vi "TypeCheck.vi"(11 "Variant in":variant) -> (2 "DbType":i32, 3 "Variant out":variant)   [LabVIEW 2020, in "ORM.lvlib" / "DbConnection.lvclass"]
uses:
  DbConnection.lvclass
  <vilib>/regexp/Match Regular Expression.xnode
  DbConnection.lvclass/DbConnection.ctl
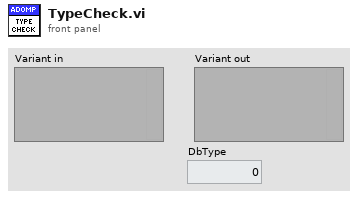
[diagram p1: front panel]
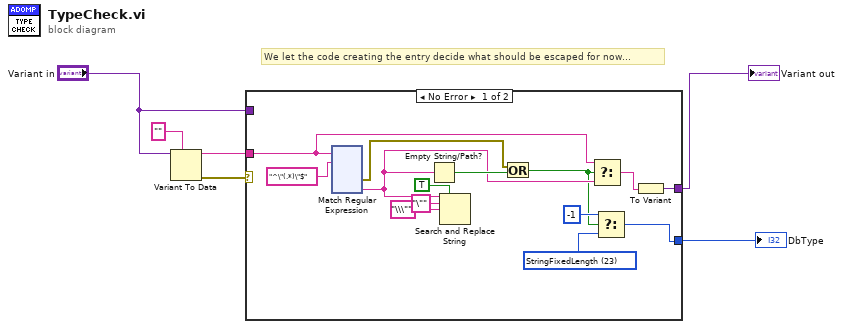
[diagram p0: block diagram]
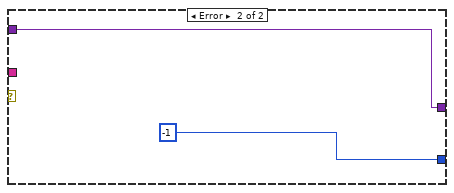
[diagram p2: hidden frame]
diagram:
  # "We let the code creating the entry decide what should be escaped for now..."
  n1 = Variant To Data(type="", Variant="Variant in") -> (data=w4:string, error out=w5:errorcluster)  [unwired: 1 in]
  n2 = case shown="No Error" w5 {
    tunnel: w4 -> [w18 _]
    tunnel: [w19 w138] -> w3
    tunnel: "Variant in" -> [_ w138]
    tunnel: [w14 -1 ("DbType")] -> w1
    frame No Error {
      w15 = 23 items=["AnsiString"=0, "Binary"=1, "Byte"=2, "Boolean"=3, "Currency"=4, "Date"=5, "DateTime"=6, "Decimal"=7, "Double"=8, "Guid"=9, "Int16"=10, "Int32"=11, "Int64"=12, "Object"=13, "SByte"=14, "Single"=15, "String"=16, "Time"=17, "UInt16"=18, "UInt32"=19, "UInt64"=20, "VarNumeric"=21, "AnsiStringFixedLength"=22, "StringFixedLength"=23, "Xml"=25, "DateTime2"=26, "DateTimeOffset"=27] ("DbType")
      n3 = xnode "Match Regular Expression"("input string"=w18, "regular expression"="^\"(.*)\"$") -> ("error out"=w7:errorcluster, "submatch 1"=w9:string)  [unwired: 4 in, 4 out]
      n4 = Empty String/Path?(string/path=w9) -> (empty?=w16:bool)
      n5 = Search and Replace String(replace all?=TRUE ("replace all? (F)"), input string=w9, search string="\"", replace string="\\\"" ("replace string (\"\")")) -> ()  [unwired: 4 in, 4 out]
      n6 = Or(x=w7, y=w16) -> (x .or. y?=w8:bool)
      n7 = Select(t=w18, s=w8, f=w9) -> (s? t:f=w17:string)
      n8 = Select(t=-1, s=w8, f=w15) -> (s? t:f=w14:i32)
      n9 = To Variant(anything=w17) -> (Variant=w19:variant)
    }
    frame Error {
    }
  }
  "Variant out" <- w3
  "DbType" <- w1
